vi "create.TradeLong.vi"(8 "error in (no error)":errorcluster, 11 "TradeLong.Parms":T1={"Time Offset"=447000, "Order Id"="ORID0001", "Execution Id"="EXE_ID_1", "Quantity"=20000, "Price"=0.905, "Side Indicator"="B", "Symbol"="AAPL"}) -> (0 "error out":errorcluster, 2 "Bytes.out":u8[](array[numeric]) format="%.0x", 3 "MessageBase out":refnum<class "TradeLong.lvclass">)   [LabVIEW 2020]
uses:
  Trade/TradeLong.Parameters.ctl
  Trade/TradeLong.lvclass
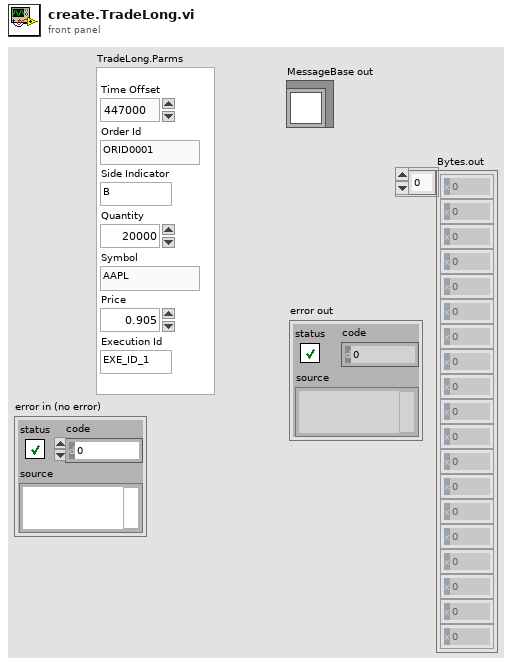
[diagram p1: front panel]
types:
  T1 = typedef "TradeLong.lvclass/TradeLong.Parameters.ctl" = cluster{"Time Offset":u32, "Order Id":string, "Execution Id":string, "Quantity":u32, "Price":dbl, "Side Indicator":string, "Symbol":string}
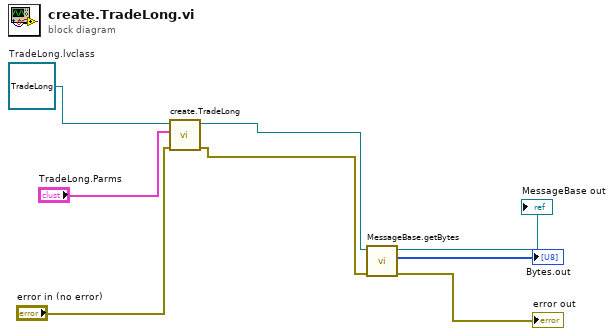
[diagram p0: block diagram]
diagram:
  w6 = refnum<class "TradeLong.lvclass"> refnum  # TradeLong.lvclass
  n1 = call-dynamic "create.TradeLong.vi"("error in"="error in (no error)", "TradeLong.Parameters"="TradeLong.Parms", "TradeLong in"=w6) -> ("error out"=w3:errorcluster, "TradeLong out"=w4:refnum<class "TradeLong.lvclass">)  [unwired: 7 in]
  n2 = call-dynamic "MessageBase.getBytes.vi"("error in (no error)"=w3, "MessageBase in"=w4) -> ("error out"=→"error out":errorcluster, "Bytes.out"=→"Bytes.out":u8[], "MessageBase out"=→"MessageBase out":refnum<class "TradeLong.lvclass">)  [unwired: 7 in]
